vi "Module Top Level.vi"(8 "error in":errorcluster, 10 "FPGA VI Reference in":T1) -> ()   [LabVIEW 2018, in "Outputs.lvlib"]
doc: "This is the top level VI for this module. It uses a queue for communications and is stopped user a user event. The general architecture is similar to a simple queued message handler.\n\nThe VIs associated with this module are organized in a LabVIEW Library."
uses:
  Outputs.lvlib
  FPGA/FPGA VI Reference.ctl
  Private Controls/Module Data.ctl
  Private Controls/Module Action.ctl
  Modules/Testing UI 1/Private Controls/APU & ECU Controls.ctl
  Modules/Testing UI 1/Public Controls/Bleed-Fuel-ECS Controls.ctl
  Public Controls/Specific Boolean Channel Write Data.ctl
  Modules/Testing UI 1/Testing UI 1.lvlib
panel:
  # "RT - Instrument IO"
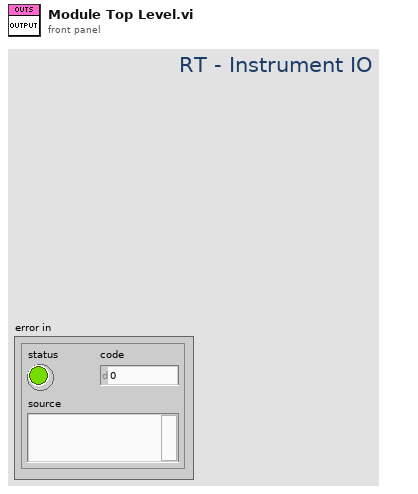
[diagram p1: front panel]
types:
  T1 = typedef "FPGA VI Reference.ctl" = refnum<k20>
  T2 = typedef "Testing UI 1.lvlib/APU & ECU Controls.ctl" = cluster{"02.01.9485.06":bool, "FuelPump":bool, "02.00.9485.01":bool, "02.00.9485.02":bool, "02.00.9485.03":bool, "02.00.9485.05":bool, "02.00.9485.04":bool, "02.00.9485.00":bool, "02.00.9485.07":bool, "02.01.9485.00":bool, "02.01.9485.01":bool}
  T3 = typedef "Testing UI 1.lvlib/Bleed-Fuel-ECS Controls.ctl" = cluster{"Coarse_RC":bool, "Coarse_RO":bool, "Bleed-Fine-Knob":dbl, "Bleed-Coarse-Knob":dbl}
  T4 = typedef "Outputs.lvlib/Specific Boolean Channel Write Data.ctl" = cluster{"Channel Index":i32, "Value":bool}
  T5 = typedef "Outputs.lvlib/Module Data.ctl" = cluster{"Data":variant, "Action":T6}
  T6 = typedef "Outputs.lvlib/Module Action.ctl" = enum16{"Init", "Error", "Write 02-06-9265 Vals (AO)", "Write 02-01-9485 Vals (DO)", "Set APU&ECU Cntrls", "Set Bleed-Fuel-ECS Cntrls", "Set ECS Demnd Cluster", "Set Fuel Pres Regltr", "Write Single 02-00-9485 Chann", "Write Single 02-01-9485 Chann"}
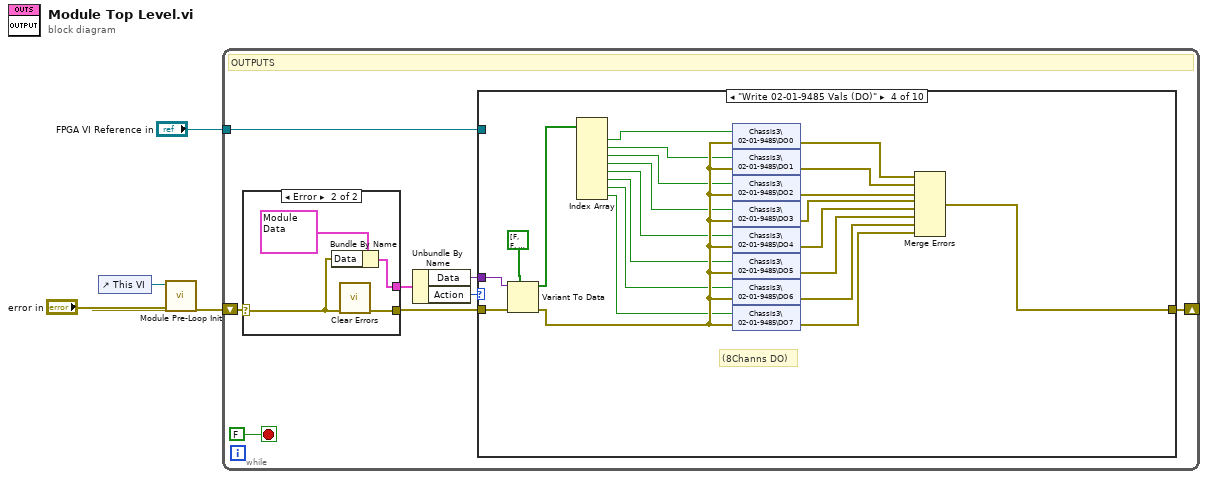
[diagram p0: block diagram]
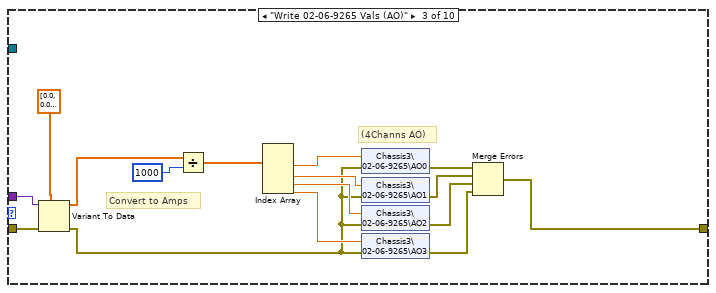
[diagram p4: hidden frame]
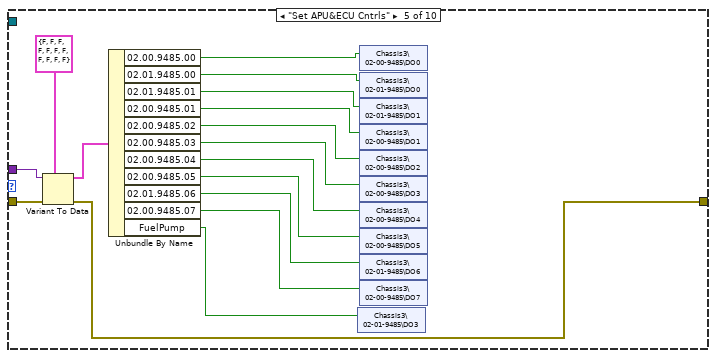
[diagram p5: hidden frame]
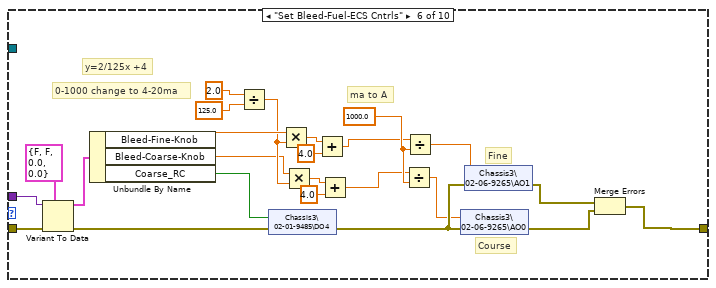
[diagram p6: hidden frame]
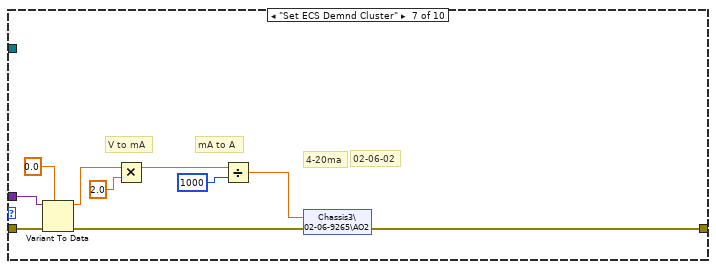
[diagram p7: hidden frame]
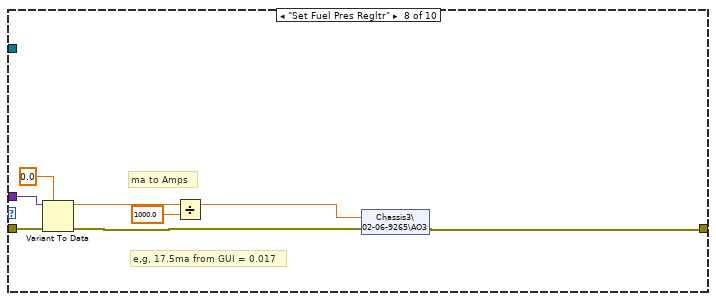
[diagram p8: hidden frame]
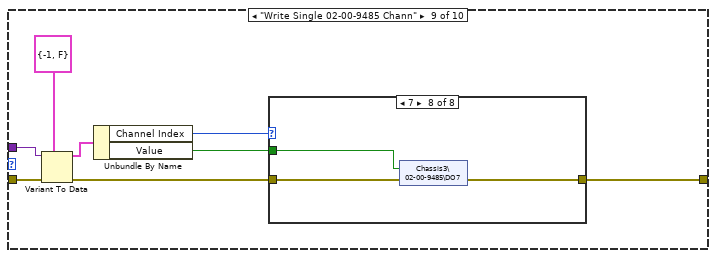
[diagram p9: hidden frame]
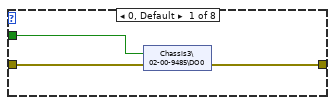
[diagram p10: hidden frame]
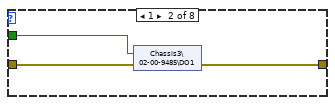
[diagram p11: hidden frame]
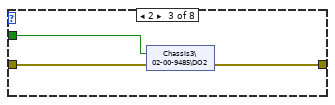
[diagram p12: hidden frame]
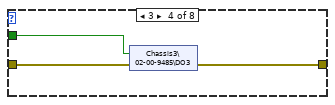
[diagram p13: hidden frame]
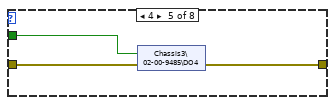
[diagram p14: hidden frame]
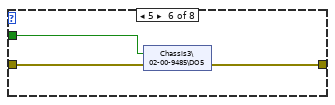
[diagram p15: hidden frame]
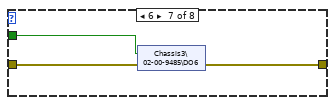
[diagram p16: hidden frame]
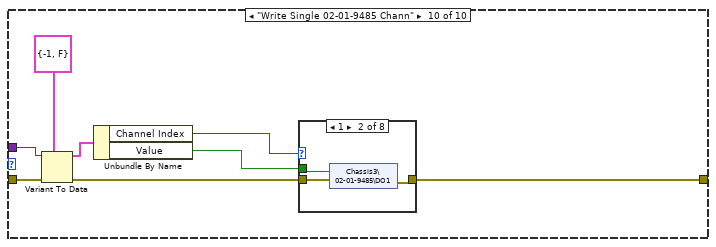
[diagram p17: hidden frame]
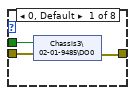
[diagram p18: hidden frame]
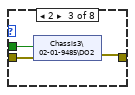
[diagram p19: hidden frame]
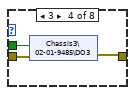
[diagram p20: hidden frame]
diagram:
  n1 = control-ref of="This VI"() -> (w4:refnum<vi>)
  n2 = call "Module Pre-Loop Init.vi"("error in (no error)"="error in", "Top Level VI Ref in"=w4) -> ("error out"=w1:errorcluster)  [unwired: 9 in]
  n3 = while {
    shift-right: [w8] -> _
    shift-left: w1 -> [w7]
    tunnel: "FPGA VI Reference in" -> [w5]
    stop <- FALSE stop-if-true
    # "OUTPUTS"
    n4 = case shown="Error" w7 {
      selector: w7 -> [w176 w179]
      tunnel: [w177 w180] -> w12
      tunnel: [w175 w178] -> w9
      frame No Error {
        n5 = call "Queue Comms Dequeue.vi"("error in (no error)"=w176) -> ("error out"=w175:errorcluster, "element"=w177:T5)  [unwired: 9 in]
      }
      frame Error {
        n6 = Bundle By Name(cluster=T5 {"Data"=variant, "Action"=enum."Error"} ("element"), "Data"=w179) -> (w180:T5)
        n7 = call <vilib>:"Clear Errors.vi"("error in (no error)"=w179) -> ("error out"=w178:errorcluster)  [unwired: 5 in, 1 out]
      }
    }
    n8 = Unbundle By Name(w12) -> ("Data"=w10:variant, "Action"=w11:T6)
    n9 = case shown="\"Write 02-01-9485 Vals (DO)\"" w11 {
      tunnel: w10 -> [_ _ w29 w51 w67 w91 w101 w109 w117 w149]
      tunnel: w9 -> [w13 w14 w30 w52 w68 w92 w102 w110 w118 w150]
      tunnel: [w13 w14 w15 w49 w55 w86 w98 w103 w111 w143] -> w8
      tunnel: w5 -> [_ _ _ _ _ _ _ _ _ _]
      frame "Init" {
      }
      frame "Error" {
      }
      frame "Write 02-06-9265 Vals (AO)" {
        # "(4Channs AO)"
        # "Convert to Amps"
        n10 = Variant To Data(error in=w30, type=dbl[] [0.0, 0.0, 0.0, 0.0], Variant=w29) -> (data=w26:dbl[], error out=w20:errorcluster)
        n11 = Divide(x=w26, y=1000 ("Numeric")) -> (x/y=w25:dbl[])
        n12 = Index Array(array=w25) -> (element #1=w24:dbl, element #2=w23:dbl, element #3=w22:dbl, element #4=w21:dbl)  [unwired: 4 in]
        n13 = shared-variable "Chassis3\\02-06-9265\\AO0"(w24, error in=w20) -> (error out=w19:errorcluster)
        n14 = shared-variable "Chassis3\\02-06-9265\\AO1"(w23, error in=w20) -> (error out=w18:errorcluster)
        n15 = shared-variable "Chassis3\\02-06-9265\\AO2"(w22, error in=w20) -> (error out=w17:errorcluster)
        n16 = shared-variable "Chassis3\\02-06-9265\\AO3"(w21, error in=w20) -> (error out=w16:errorcluster)
        n17 = Merge Errors(w19, w18, w17, w16) -> (w15:errorcluster)
      }
      frame "Write 02-01-9485 Vals (DO)" {
        # "(8Channs DO)"
        n18 = Variant To Data(error in=w52, type=bool[] [FALSE, FALSE, FALSE, FALSE, FALSE, FALSE, FALSE, FALSE], Variant=w51) -> (data=w48:bool[], error out=w47:errorcluster)
        n19 = Index Array(array=w48) -> (element #1=w38:bool, element #2=w37:bool, element #3=w36:bool, element #4=w35:bool, element #5=w34:bool, element #6=w33:bool, element #7=w32:bool, element #8=w31:bool)  [unwired: 8 in]
        n20 = shared-variable "Chassis3\\02-01-9485\\DO0"(w38, error in=w47) -> (error out=w46:errorcluster)
        n21 = shared-variable "Chassis3\\02-01-9485\\DO1"(w37, error in=w47) -> (error out=w45:errorcluster)
        n22 = shared-variable "Chassis3\\02-01-9485\\DO2"(w36, error in=w47) -> (error out=w44:errorcluster)
        n23 = shared-variable "Chassis3\\02-01-9485\\DO3"(w35, error in=w47) -> (error out=w43:errorcluster)
        n24 = shared-variable "Chassis3\\02-01-9485\\DO4"(w34, error in=w47) -> (error out=w42:errorcluster)
        n25 = shared-variable "Chassis3\\02-01-9485\\DO5"(w33, error in=w47) -> (error out=w41:errorcluster)
        n26 = shared-variable "Chassis3\\02-01-9485\\DO6"(w32, error in=w47) -> (error out=w40:errorcluster)
        n27 = shared-variable "Chassis3\\02-01-9485\\DO7"(w31, error in=w47) -> (error out=w39:errorcluster)
        n28 = Merge Errors(w46, w45, w44, w43, w42, w41, w40, w39) -> (w49:errorcluster)
      }
      frame "Set APU&ECU Cntrls" {
        n29 = Variant To Data(error in=w68, type=T2 {"02.01.9485.06"=FALSE, "FuelPump"=FALSE, "02.00.9485.01"=FALSE, "02.00.9485.02"=FALSE, "02.00.9485.03"=FALSE, "02.00.9485.05"=FALSE, "02.00.9485.04"=FALSE, "02.00.9485.00"=FALSE, "02.00.9485.07"=FALSE, "02.01.9485.00"=FALSE, "02.01.9485.01"=FALSE} ("APU & ECU Controls"), Variant=w67) -> (data=w65:T2, error out=w55:errorcluster)
        n30 = Unbundle By Name(w65) -> ("02.00.9485.00"=w64:bool, "02.01.9485.00"=w63:bool, "02.01.9485.01"=w62:bool, "02.00.9485.01"=w54:bool, "02.00.9485.02"=w61:bool, "02.00.9485.03"=w60:bool, "02.00.9485.04"=w59:bool, "02.00.9485.05"=w58:bool, "02.01.9485.06"=w57:bool, "02.00.9485.07"=w56:bool, "FuelPump"=w53:bool)
        n31 = shared-variable "Chassis3\\02-01-9485\\DO3"(w53) -> ()  [unwired: 1 in, 1 out]
        n32 = shared-variable "Chassis3\\02-00-9485\\DO0"(w64) -> ()  [unwired: 1 in, 1 out]
        n33 = shared-variable "Chassis3\\02-01-9485\\DO0"(w63) -> ()  [unwired: 1 in, 1 out]
        n34 = shared-variable "Chassis3\\02-01-9485\\DO1"(w62) -> ()  [unwired: 1 in, 1 out]
        n35 = shared-variable "Chassis3\\02-00-9485\\DO1"(w54) -> ()  [unwired: 1 in, 1 out]
        n36 = shared-variable "Chassis3\\02-00-9485\\DO2"(w61) -> ()  [unwired: 1 in, 1 out]
        n37 = shared-variable "Chassis3\\02-00-9485\\DO3"(w60) -> ()  [unwired: 1 in, 1 out]
        n38 = shared-variable "Chassis3\\02-00-9485\\DO4"(w59) -> ()  [unwired: 1 in, 1 out]
        n39 = shared-variable "Chassis3\\02-00-9485\\DO5"(w58) -> ()  [unwired: 1 in, 1 out]
        n40 = shared-variable "Chassis3\\02-01-9485\\DO6"(w57) -> ()  [unwired: 1 in, 1 out]
        n41 = shared-variable "Chassis3\\02-00-9485\\DO7"(w56) -> ()  [unwired: 1 in, 1 out]
      }
      frame "Set Bleed-Fuel-ECS Cntrls" {
        w84 = 1000.0 ("y")
        # "y=2/125x +4"
        # "ma to A"
        # "0-1000 change to 4-20ma"
        # "Fine"
        # "Course"
        n42 = Variant To Data(error in=w92, type=T3 {"Coarse_RC"=FALSE, "Coarse_RO"=FALSE, "Bleed-Fine-Knob"=0.0, "Bleed-Coarse-Knob"=0.0} ("Bleed-Fuel-ECS Controls"), Variant=w91) -> (data=w89:T3, error out=w88:errorcluster)
        n43 = Unbundle By Name(w89) -> ("Bleed-Fine-Knob"=w79:dbl, "Bleed-Coarse-Knob"=w70:dbl, "Coarse_RC"=w80:bool)
        n44 = Divide(x=2.0 ("y"), y=125.0) -> (x/y=w71:dbl)
        n45 = shared-variable "Chassis3\\02-01-9485\\DO4"(w80, error in=w88) -> (error out=w87:errorcluster)
        n46 = Multiply(x=w79, y=w71) -> (x*y=w76:dbl)
        n47 = Multiply(x=w70, y=w71) -> (x*y=w73:dbl)
        n48 = Add(x=w76, y=4.0) -> (x+y=w74:dbl)
        n49 = Add(x=w73, y=4.0) -> (x+y=w69:dbl)
        n50 = Divide(x=w69, y=w84) -> (x/y=w83:dbl)
        n51 = Divide(x=w74, y=w84) -> (x/y=w85:dbl)
        n52 = shared-variable "Chassis3\\02-06-9265\\AO0"(w83, error in=w87) -> (error out=w81:errorcluster)
        n53 = shared-variable "Chassis3\\02-06-9265\\AO1"(w85, error in=w87) -> (error out=w82:errorcluster)
        n54 = Merge Errors(w82, w81) -> (w86:errorcluster)
      }
      frame "Set ECS Demnd Cluster" {
        # "mA to A"
        # "V to mA"
        # "4-20ma"
        # "02-06-02"
        n55 = Variant To Data(error in=w102, type=0.0, Variant=w101) -> (data=w96:dbl, error out=w99:errorcluster)
        n56 = Multiply(x=w96, y=2.0) -> (x*y=w94:dbl)
        n57 = Divide(x=w94, y=1000 ("Numeric")) -> (x/y=w95:dbl)
        n58 = shared-variable "Chassis3\\02-06-9265\\AO2"(w95, error in=w99) -> (error out=w98:errorcluster)
      }
      frame "Set Fuel Pres Regltr" {
        # "e,g, 17.5ma from GUI = 0.017"
        # "ma to Amps"
        n59 = Variant To Data(error in=w110, type=0.0, Variant=w109) -> (data=w107:dbl, error out=w104:errorcluster)
        n60 = Divide(x=w107, y=1000.0) -> (x/y=w105:dbl)
        n61 = shared-variable "Chassis3\\02-06-9265\\AO3"(w105, error in=w104) -> (error out=w103:errorcluster)
      }
      frame "Write Single 02-00-9485 Chann" {
        n62 = Variant To Data(error in=w118, type=T4 {"Channel Index"=-1, "Value"=FALSE} ("Chann and Val"), Variant=w117) -> (data=w115:T4, error out=w112:errorcluster)
        n63 = Unbundle By Name(w115) -> ("Channel Index"=w114:i32, "Value"=w113:bool)
        n64 = case shown="7" w114 {
          tunnel: w113 -> [w121 w123 w126 w130 w133 w136 w138 w141]
          tunnel: w112 -> [w120 w124 w127 w129 w132 w135 w139 w142]
          tunnel: [w119 w122 w125 w128 w131 w134 w137 w140] -> w111
          frame 0, Default {
            n65 = shared-variable "Chassis3\\02-00-9485\\DO0"(w121, error in=w120) -> (error out=w119:errorcluster)
          }
          frame 1 {
            n66 = shared-variable "Chassis3\\02-00-9485\\DO1"(w123, error in=w124) -> (error out=w122:errorcluster)
          }
          frame 2 {
            n67 = shared-variable "Chassis3\\02-00-9485\\DO2"(w126, error in=w127) -> (error out=w125:errorcluster)
          }
          frame 3 {
            n68 = shared-variable "Chassis3\\02-00-9485\\DO3"(w130, error in=w129) -> (error out=w128:errorcluster)
          }
          frame 4 {
            n69 = shared-variable "Chassis3\\02-00-9485\\DO4"(w133, error in=w132) -> (error out=w131:errorcluster)
          }
          frame 5 {
            n70 = shared-variable "Chassis3\\02-00-9485\\DO5"(w136, error in=w135) -> (error out=w134:errorcluster)
          }
          frame 6 {
            n71 = shared-variable "Chassis3\\02-00-9485\\DO6"(w138, error in=w139) -> (error out=w137:errorcluster)
          }
          frame 7 {
            n72 = shared-variable "Chassis3\\02-00-9485\\DO7"(w141, error in=w142) -> (error out=w140:errorcluster)
          }
        }
      }
      frame "Write Single 02-01-9485 Chann" {
        n73 = Variant To Data(error in=w150, type=T4 {"Channel Index"=-1, "Value"=FALSE} ("Chann and Val"), Variant=w149) -> (data=w147:T4, error out=w144:errorcluster)
        n74 = Unbundle By Name(w147) -> ("Channel Index"=w146:i32, "Value"=w145:bool)
        n75 = case shown="1" w146 {
          tunnel: w145 -> [w152 w155 w158 w161 w164 w167 w170 w173]
          tunnel: w144 -> [w153 w156 w159 w162 w165 w168 w171 w174]
          tunnel: [w151 w154 w157 w160 w163 w166 w169 w172] -> w143
          frame 0, Default {
            n76 = shared-variable "Chassis3\\02-01-9485\\DO0"(w152, error in=w153) -> (error out=w151:errorcluster)
          }
          frame 1 {
            n77 = shared-variable "Chassis3\\02-01-9485\\DO1"(w155, error in=w156) -> (error out=w154:errorcluster)
          }
          frame 2 {
            n78 = shared-variable "Chassis3\\02-01-9485\\DO2"(w158, error in=w159) -> (error out=w157:errorcluster)
          }
          frame 3 {
            n79 = shared-variable "Chassis3\\02-01-9485\\DO3"(w161, error in=w162) -> (error out=w160:errorcluster)
          }
          frame 4 {
            n80 = shared-variable "Chassis3\\02-01-9485\\DO4"(w164, error in=w165) -> (error out=w163:errorcluster)
          }
          frame 5 {
            n81 = shared-variable "Chassis3\\02-01-9485\\DO5"(w167, error in=w168) -> (error out=w166:errorcluster)
          }
          frame 6 {
            n82 = shared-variable "Chassis3\\02-01-9485\\DO6"(w170, error in=w171) -> (error out=w169:errorcluster)
          }
          frame 7 {
            n83 = shared-variable "Chassis3\\02-01-9485\\DO7"(w173, error in=w174) -> (error out=w172:errorcluster)
          }
        }
      }
    }
  }
